vi "Test Stopwatch.vi"(11 "Error in":errorcluster) -> (15 "Error out":errorcluster)   [LabVIEW 2020, in "StopWatchTests.lvlib"]
doc: "This VI is used for validating stopwatch"
uses:
  StopWatchTests.lvlib
  <vilib>/addons/_JKI Toolkits/Caraya/classes/Test Suite/Define Test Suite (JUnit Report).vi
  <vilib>/SLL Drona/APIs/Stimulus/ControlValue/SetValueAuto.vi
  <vilib>/SLL Drona/APIs/Assert/AssertControlValue/AlmostEqual.vi
  <vilib>/SLL Drona/APIs/Assert/AssertControlValue/Equal.vi
  <vilib>/SLL Drona/APIs/Stimulus/VI/CloseVI.vi
  <vilib>/Utility/error.llb/Error Cluster From Error Code.vi
  <vilib>/ErrorRing/Error Ring.xnode
  <vilib>/addons/_JKI Toolkits/Caraya/classes/Test Suite/Test Suite.lvclass
  <vilib>/addons/_JKI Toolkits/Caraya/classes/Test/Test.lvclass
  <vilib>/SLL Drona/Drona.lvlib
  <vilib>/SLL Drona/APIs/Stimulus/ControlValue/ControlValue.lvlib
  <vilib>/SLL Drona/APIs/Assert/AssertControlValue/AssertControlValue.lvlib
  <vilib>/Wiresmith Technology/G CLI/CLI Class/CLI.lvclass
  <vilib>/SLL Drona/APIs/Stimulus/VI/VI.lvlib
panel:
  # "STOPWATCH TEST"
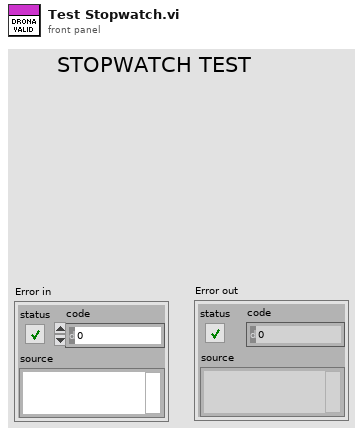
[diagram p1: front panel]
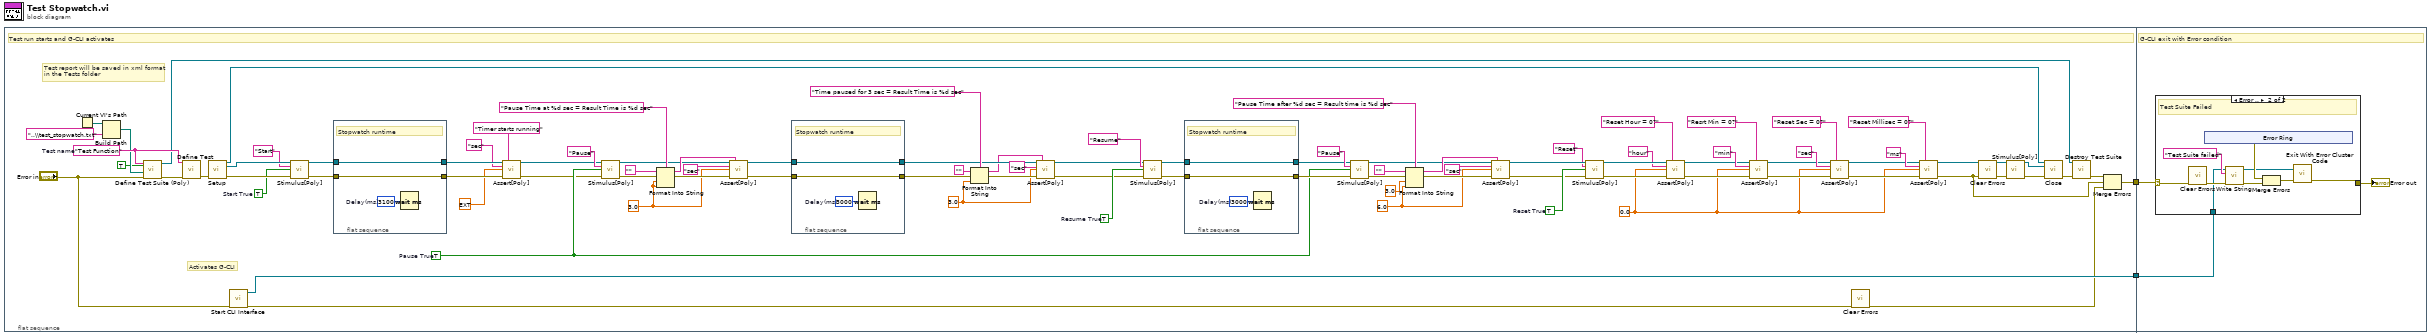
[diagram p0: block diagram]
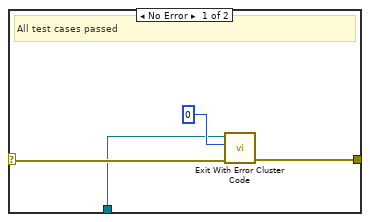
[diagram p2: hidden frame]
diagram:
  n1 = flat-sequence {
    tunnel: [w6] -> w2
    tunnel: [w3] -> w1
    tunnel: w2 -> [w106]
    tunnel: w1 -> [w107]
    frame #0 {
      w30 = 3.0 ("input 1")
      w44 = 0.0 ("input 1")
      w65 = TRUE  # Reset True
      w67 = 6.0 ("input 1")
      w80 = TRUE  # Resume True
      w68 = 3.0 ("input 1")
      w62 = TRUE  # Pause True
      w90 = TRUE  # Start True
      w17 = "Test Function"  # Test name
      # "Activates G-CLI"
      # "Test report will be saved in xml format\nin the Tests folder"
      # "Test run starts and G-CLI activates"
      n2 = Current VI's Path() -> (path=w16:path)
      n3 = Build Path(base path=w16, name or relative path="..\\test_stopwatch.txt") -> (appended path=w14:path)
      n4 = call-poly <vilib>:"Define Test Suite (Poly).vi"("error in (no error)"="Error in", "Report Path"=w14, "Interactive"=TRUE, "Label (VI Title)"=w17) -> ("error out"=w18:errorcluster, "Test Suite"=w4:refnum<class "Test Suite.lvclass">)  [unwired: 5 in, 1 out]
      n5 = call <vilib>:"Define Test.vi"("error in (no error)"=w18, "Label (VI Title)"=w17) -> ("error out"=w95:errorcluster)  [unwired: 8 in, 1 out]
      n6 = call <vilib>:"Setup.vi"("error in"=w95) -> ("Application Ref"=w92:refnum<vi>, "VI Reference Out"=w93:refnum<vi>, "error out"=w94:errorcluster)  [unwired: 12 in]
      n7 = call <vilib>:"Start CLI Interface.vi"("error in (no error)"="Error in") -> ("error out"=w7:errorcluster, "CLI out"=w6:refnum<class "CLI.lvclass">)  [unwired: 7 in, 2 out]
      n8 = call-poly <vilib>:"Stimulus[Poly].vi"("VI Reference In"=w93, "Control Path"="Start", "Value (Signaling)"=w90, "error in"=w94) -> ("VI Reference Out"=w87:refnum<vi>, "error out"=w89:errorcluster)  [unwired: 10 in]
      n9 = flat-sequence {
        tunnel: w89 -> [w104]
        tunnel: [w104] -> w25
        tunnel: [w102] -> w24
        tunnel: w87 -> [w102]
        frame #0 {
          w103 = u32 3100  # Delay(ms)
          # "Stopwatch runtime"
          n10 = Wait (ms)(milliseconds to wait=w103) -> ()  [unwired: 1 out]
        }
      }
      n11 = call-poly <vilib>:"Assert[Poly].vi"("VI Reference In"=w24, "Test Label"="Timer starts running", "Control Path"="sec", "Control Value"=ext 3.0, "Error In"=w25) -> ("VI Reference Out"=w21:refnum<vi>, "Error Out"=w20:errorcluster)  [unwired: 9 in]
      n12 = call-poly <vilib>:"Stimulus[Poly].vi"("VI Reference In"=w21, "Control Path"="Pause", "Value (Signaling)"=w62, "error in"=w20) -> ("VI Reference Out"=w42:refnum<vi>, "error out"=w86:errorcluster)  [unwired: 10 in]
      n13 = Format Into String(format string="Pause Time at %d sec = Result Time is %d sec", initial string="", error in=w86, w68, w68) -> (resulting string=w83:string, error out=w85:errorcluster)
      n14 = call-poly <vilib>:"Assert[Poly].vi"("VI Reference In"=w42, "Test Label"=w83, "Control Path"="sec", "Control Value"=w68, "Error In"=w85) -> ("VI Reference Out"=w41:refnum<vi>, "Error Out"=w40:errorcluster)  [unwired: 9 in]
      n15 = flat-sequence {
        tunnel: w40 -> [w98]
        tunnel: [w98] -> w39
        tunnel: [w96] -> w35
        tunnel: w41 -> [w96]
        frame #0 {
          w97 = u32 3000  # Delay(ms)
          # "Stopwatch runtime"
          n16 = Wait (ms)(milliseconds to wait=w97) -> ()  [unwired: 1 out]
        }
      }
      n17 = Format Into String(format string="Time paused for 3 sec = Result Time is %d sec", initial string="", error in=w39, w30) -> (resulting string=w32:string, error out=w36:errorcluster)
      n18 = call-poly <vilib>:"Assert[Poly].vi"("VI Reference In"=w35, "Test Label"=w32, "Control Path"="sec", "Control Value"=w30, "Error In"=w36) -> ("VI Reference Out"=w33:refnum<vi>, "Error Out"=w34:errorcluster)  [unwired: 9 in]
      n19 = call-poly <vilib>:"Stimulus[Poly].vi"("VI Reference In"=w33, "Control Path"="Resume", "Value (Signaling)"=w80, "error in"=w34) -> ("VI Reference Out"=w78:refnum<vi>, "error out"=w79:errorcluster)  [unwired: 10 in]
      n20 = flat-sequence {
        tunnel: w79 -> [w101]
        tunnel: [w101] -> w72
        tunnel: [w99] -> w73
        tunnel: w78 -> [w99]
        frame #0 {
          w100 = u32 3000  # Delay(ms)
          # "Stopwatch runtime"
          n21 = Wait (ms)(milliseconds to wait=w100) -> ()  [unwired: 1 out]
        }
      }
      n22 = call-poly <vilib>:"Stimulus[Poly].vi"("VI Reference In"=w73, "Control Path"="Pause", "Value (Signaling)"=w62, "error in"=w72) -> ("VI Reference Out"=w66:refnum<vi>, "error out"=w75:errorcluster)  [unwired: 10 in]
      n23 = Format Into String(format string="Pause Time after %d sec = Result time is %d sec", initial string="", error in=w75, 3.0 ("input 2"), w67) -> (resulting string=w69:string, error out=w70:errorcluster)
      n24 = call-poly <vilib>:"Assert[Poly].vi"("VI Reference In"=w66, "Test Label"=w69, "Control Path"="sec", "Control Value"=w67, "Error In"=w70) -> ("VI Reference Out"=w63:refnum<vi>, "Error Out"=w64:errorcluster)  [unwired: 9 in]
      n25 = call-poly <vilib>:"Stimulus[Poly].vi"("VI Reference In"=w63, "Control Path"="Reset", "Value (Signaling)"=w65, "error in"=w64) -> ("VI Reference Out"=w58:refnum<vi>, "error out"=w60:errorcluster)  [unwired: 10 in]
      n26 = call-poly <vilib>:"Assert[Poly].vi"("VI Reference In"=w58, "Test Label"="Reset Hour = 0?" ("Label"), "Control Path"="hour", "Control Value"=w44, "Error In"=w60) -> ("VI Reference Out"=w54:refnum<vi>, "Error Out"=w53:errorcluster)  [unwired: 9 in]
      n27 = call-poly <vilib>:"Assert[Poly].vi"("VI Reference In"=w54, "Test Label"="Resrt Min = 0?" ("Label"), "Control Path"="min", "Control Value"=w44, "Error In"=w53) -> ("VI Reference Out"=w49:refnum<vi>, "Error Out"=w50:errorcluster)  [unwired: 9 in]
      n28 = call-poly <vilib>:"Assert[Poly].vi"("VI Reference In"=w49, "Test Label"="Reset Sec = 0?" ("Label"), "Control Path"="sec", "Control Value"=w44, "Error In"=w50) -> ("VI Reference Out"=w45:refnum<vi>, "Error Out"=w46:errorcluster)  [unwired: 9 in]
      n29 = call <vilib>:"Clear Errors.vi"("error in (no error)"=w7) -> ("error out"=w5:errorcluster)  [unwired: 5 in, 1 out]
      n30 = call-poly <vilib>:"Assert[Poly].vi"("VI Reference In"=w45, "Test Label"="Reset Millisec = 0?" ("Label"), "Control Path"="ms", "Control Value"=w44, "Error In"=w46) -> ("VI Reference Out"=w28:refnum<vi>, "Error Out"=w8:errorcluster)  [unwired: 9 in]
      n31 = call <vilib>:"Clear Errors.vi"("error in (no error)"=w8) -> ("error out"=w11:errorcluster)  [unwired: 5 in, 1 out]
      n32 = call-poly <vilib>:"Stimulus[Poly].vi"("VI Reference In"=w28, "error in"=w11) -> ("VI Reference Out"=w27:refnum<vi>, "error out"=w26:errorcluster)  [unwired: 12 in]
      n33 = call <vilib>:"Close.vi"("Application Ref"=w92, "VI Reference"=w27, "error in"=w26) -> ("error out"=w10:errorcluster)  [unwired: 12 in]
      n34 = call-dynamic "Destroy Test Suite.vi"("error in (no error)"=w10, "Test Suite in"=w4) -> ("error out"=w9:errorcluster)  [unwired: 8 in, 1 out]
      n35 = Merge Errors(w9, w8, w5) -> (w3:errorcluster)
    }
    frame #1 {
      # "G-CLI exit with Error condition"
      n36 = case shown="Error .." w107 {
        selector: w107 -> [w111 w118]
        tunnel: w106 -> [w109 w113]
        tunnel: [w108 w120] -> w105
        frame No Error {
          # "All test cases passed"
          n37 = call <vilib>:"Exit With Error Cluster Code.vi"("error in (no error)"=w111, "No Error Code (0)"=0, "CLI in"=w109) -> ("error out"=w108:errorcluster)  [unwired: 8 in]
        }
        frame Error {
          # "Test Suite Failed"
          n38 = call <vilib>:"Clear Errors.vi"("error in (no error)"=w118) -> ("error out"=w117:errorcluster)  [unwired: 5 in, 1 out]
          n39 = xnode "Error Ring"() -> ("error out"=w116:errorcluster)
          n40 = call <vilib>:"Write String.vi"("error in (no error)"=w117, "Text to Write"="Test Suite failed", "CLI in"=w113) -> ("error out"=w115:errorcluster, "CLI out"=w112:refnum<class "CLI.lvclass">)  [unwired: 7 in]
          n41 = Merge Errors(w116, w115) -> (w114:errorcluster)
          n42 = call <vilib>:"Exit With Error Cluster Code.vi"("error in (no error)"=w114, "CLI in"=w112) -> ("error out"=w120:errorcluster)  [unwired: 9 in]
        }
      }
      "Error out" <- w105
    }
  }
